vi "Ctor.vi"(8 "error in (no error)":errorcluster, 11 "GWebAppArrayPanel in":refnum<class "GWebAppArrayPanel.lvclass">) -> (0 "error out":errorcluster, 3 "GWebAppArrayPanel out":refnum<class "GWebAppArrayPanel.lvclass">)   [LabVIEW 2020, in "PicoG-App.lvlib" / "GWebAppArrayPanel.lvclass"]
uses:
  GWebAppArrayPanel.lvclass
  Ref Data.ctl
  ViaApp/ViaApp.lvclass
  Outbound Events.ctl
  GWebAppArrayPanel.lvclass/GWebAppArrayPanel.ctl
  <vilib>/IlluminatedG/IG OOPanel/OOPanel/ArrayPanel/ArrayPanel.lvclass
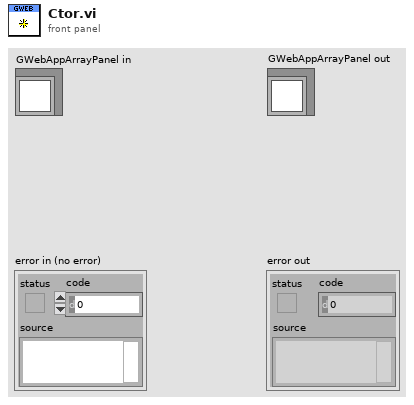
[diagram p1: front panel]
types:
  T1 = typedef "PicoG-App.lvlib/GWebAppArrayPanel.lvclass/Ref Data.ctl" = cluster{"App":refnum<class "ViaApp.lvclass">, "Outbound Events":T2}
  T2 = typedef "PicoG-App.lvlib/GWebAppArrayPanel.lvclass/Outbound Events.ctl" = cluster{"Select App":refnum<user-event>}
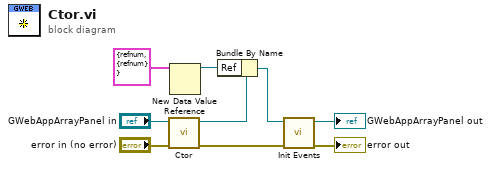
[diagram p0: block diagram]
diagram:
  n1 = call-parent "Ctor.vi"("error in (no error)"="error in (no error)", "ArrayPanel in"="GWebAppArrayPanel in") -> ("error out"=w1:errorcluster, "ArrayPanel out"=w2:refnum<class "GWebAppArrayPanel.lvclass">)  [unwired: 8 in]
  n2 = New Data Value Reference(data value=T1 {"App"=refnum, "Outbound Events"={"Select App"=refnum}} ("Ref Data")) -> (data value reference=w5:refnum<data-value>)  [unwired: 1 in, 1 out]
  n3 = Bundle By Name(cluster=w2, "Ref"=w5) -> (w6:refnum<class "GWebAppArrayPanel.lvclass">)
  n4 = call "Init Events.vi"("error in (no error)"=w1, "GWebAppArrayPanel in"=w6) -> ("error out"=→"error out":errorcluster, "GWebAppArrayPanel out"=→"GWebAppArrayPanel out":refnum<class "GWebAppArrayPanel.lvclass">)  [unwired: 8 in]
